vi "PH_Cam_BaseClass.calc Centroid Offset.vi"(2 "Resolution":i32, 7 "Centroid":dbl) -> (8 "Offset":string)   [LabVIEW 2014, in "PH_Cam_BaseClass.lvlib"]
doc: "Calculates:\n\n(((Centroid-(Resolution/2))*100)/Resolution)*2\n\nconverts the result to string and adds a \"_%\""
uses:
  PH_Cam_BaseClass.lvlib
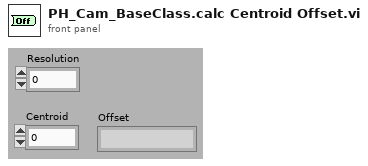
[diagram p1: front panel]
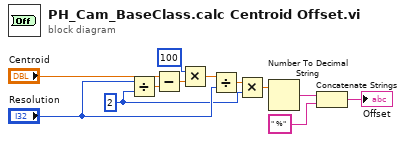
[diagram p0: block diagram]
diagram:
  w1 = 2 ("y")
  n1 = Divide(x="Resolution", y=w1) -> (x/y=w8:dbl)
  n2 = Subtract(x="Centroid", y=w8) -> (x-y=w9:dbl)
  n3 = Multiply(x=100 ("y"), y=w9) -> (x*y=w12:dbl)
  n4 = Divide(x=w12, y="Resolution") -> (x/y=w3:dbl)
  n5 = Multiply(x=w3, y=w1) -> (x*y=w2:dbl)
  n6 = Number To Decimal String(number=w2) -> (decimal integer string=w11:string)  [unwired: 1 in]
  n7 = Concatenate Strings(w11, " %" ("string")) -> (→"Offset":string)
